vi "GUNSC_LibSetArrangeSectionsY.vi"(8 "error in (no error)":errorcluster, 9 "how":string, 11 "Database RefNum out":T1) -> (0 "error out":errorcluster, 1 "response":string, 2 "return value":i32)   [LabVIEW 2014]
uses:
  panview/PAN/Modules/DBSHAND/private/vis/DatabaseHand_RefNum.ctl
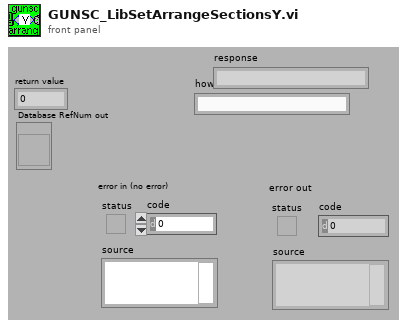
[diagram p1: front panel]
types:
  T1 = typedef "DatabaseHand_RefNum.ctl" = refnum<vi>
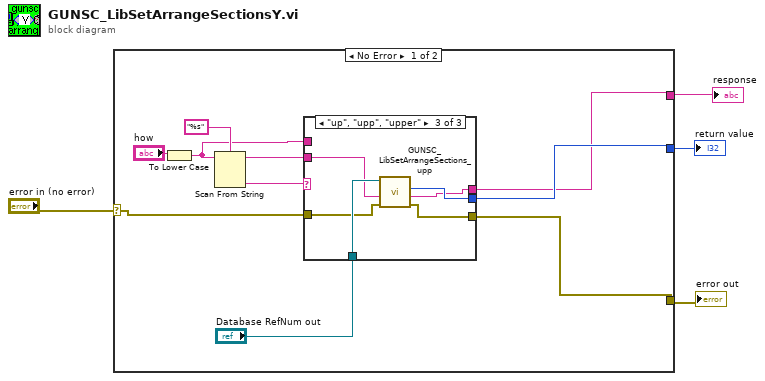
[diagram p0: block diagram]
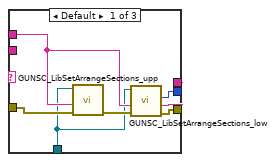
[diagram p2: hidden frame]
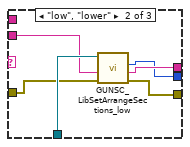
[diagram p3: hidden frame]
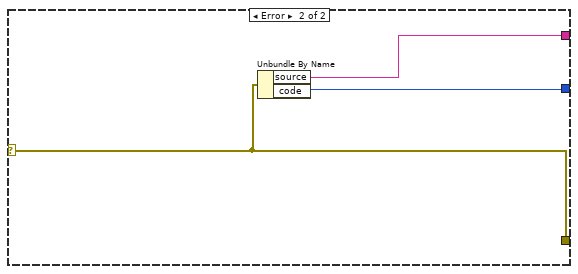
[diagram p4: hidden frame]
diagram:
  n1 = case shown="No Error" "error in (no error)" {
    selector: "error in (no error)" -> [w13 w36]
    tunnel: [w11 w35] -> w4
    tunnel: [w12 w36] -> w2
    tunnel: [w10 w34] -> w1
    frame No Error {
      n2 = To Lower Case(string="how") -> (all lower case string=w7:string)
      n3 = Scan From String(format string="%s", input string=w7) -> (remaining string=w6:string, output 1=w9:string)  [unwired: 2 in, 3 out]
      n4 = case shown="\"up\", \"upp\", \"upper\"" w9 {
        tunnel: w6 -> [_ w22 w32]
        tunnel: w13 -> [w21 w24 w28]
        tunnel: [w19 w23 w29] -> w12
        tunnel: [w18 w25 w31] -> w11
        tunnel: [w17 w26 w30] -> w10
        tunnel: w7 -> [w16 _ _]
        tunnel: "Database RefNum out" -> [w15 w27 w33]
        frame Default {
          n5 = call "GUNSC_LibSetArrangeSections_upp.vi"("error in (no error)"=w21, "how"=w16, "Database RefNum out"=w15) -> ("error out"=w20:errorcluster)  [unwired: 8 out]
          n6 = call "GUNSC_LibSetArrangeSections_low.vi"("error in (no error)"=w20, "how"=w16, "Database RefNum out"=w15) -> ("error out"=w19:errorcluster, "response"=w17:string, "return value"=w18:i32)  [unwired: 6 out]
        }
        frame "low", "lower" {
          n7 = call "GUNSC_LibSetArrangeSections_low.vi"("error in (no error)"=w24, "how"=w22, "Database RefNum out"=w27) -> ("error out"=w23:errorcluster, "response"=w26:string, "return value"=w25:i32)  [unwired: 6 out]
        }
        frame "up", "upp", "upper" {
          n8 = call "GUNSC_LibSetArrangeSections_upp.vi"("error in (no error)"=w28, "how"=w32, "Database RefNum out"=w33) -> ("error out"=w29:errorcluster, "response"=w30:string, "return value"=w31:i32)  [unwired: 6 out]
        }
      }
    }
    frame Error {
      n9 = Unbundle By Name(w36) -> ("source"=w34:string, "code"=w35:i32)
    }
  }
  "return value" <- w4
  "error out" <- w2
  "response" <- w1
